vi "PixelClockU32._N5771_Resonance.vi"(10 "Samples per pixel":u32=16960, 11 "Sample counter":u32=16960) -> (3 "Pixel clock":bool)   [LabVIEW 2012]
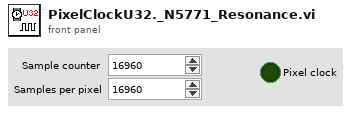
[diagram p1: front panel]
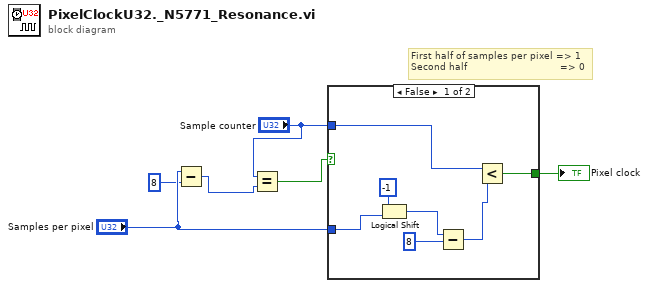
[diagram p0: block diagram]
diagram:
  # "First half of samples per pixel => 1\nSecond half                               => 0"
  n1 = Subtract(x="Samples per pixel", y=u32 8) -> (x-y=w4:u32)
  n2 = Equal?(x="Sample counter", y=w4) -> (x = y?=w5:bool)
  n3 = case shown="False" w5 {
    selector: w5 -> [_ w14]
    tunnel: "Samples per pixel" -> [w13 _]
    tunnel: "Sample counter" -> [w11 _]
    tunnel: [w10 w14] -> w6
    frame False {
      n4 = Logical Shift(y=i16 -1, x=w13) -> (x << y=w9:u32)
      n5 = Subtract(x=w9, y=u32 8) -> (x-y=w8:u32)
      n6 = Less?(x=w11, y=w8) -> (x < y?=w10:bool)
    }
    frame True {
    }
  }
  "Pixel clock" <- w6
